vi "Get ROI Description String.vi"(8 "Error In":errorcluster, 9 "Contours":T2(array[cluster]), 11 "Global Rectangle":i32[](array[numeric])) -> (0 "Error Out":errorcluster, 3 "ROI Description String":string)   [LabVIEW 2021, in "Image.lvlib"]
uses:
  Image.lvlib
  Image ROI Type.ctl
  Math/Math.lvlib
  Strings/Strings.lvlib
panel:
  in  "Type":T1
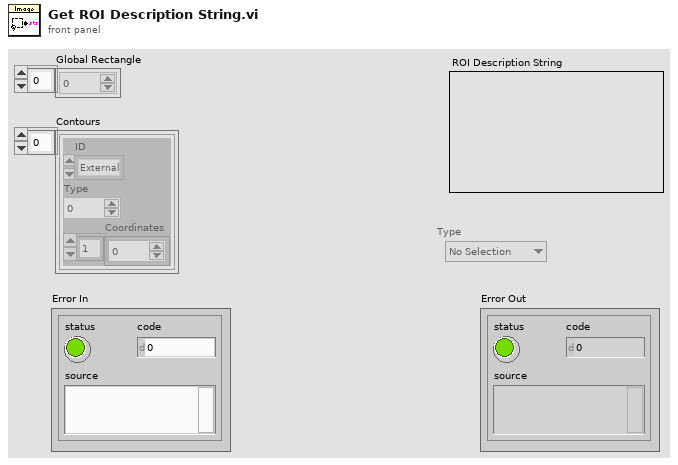
[diagram p1: front panel]
types:
  T1 = typedef "Image.lvlib/Image ROI Type.ctl" = enum16{"No Selection", "Point", "Line", "Rectangle", "Oval", "Polygon", "Freehand Region", "Annulus", "Unused2", "Unused3", "Broken Line", "Freehand Line", "Rotated Rectangle"}
  T2 = cluster{"ID":enum32{"External", "Internal"}, "Type":u32, "Coordinates":i32[]}[]
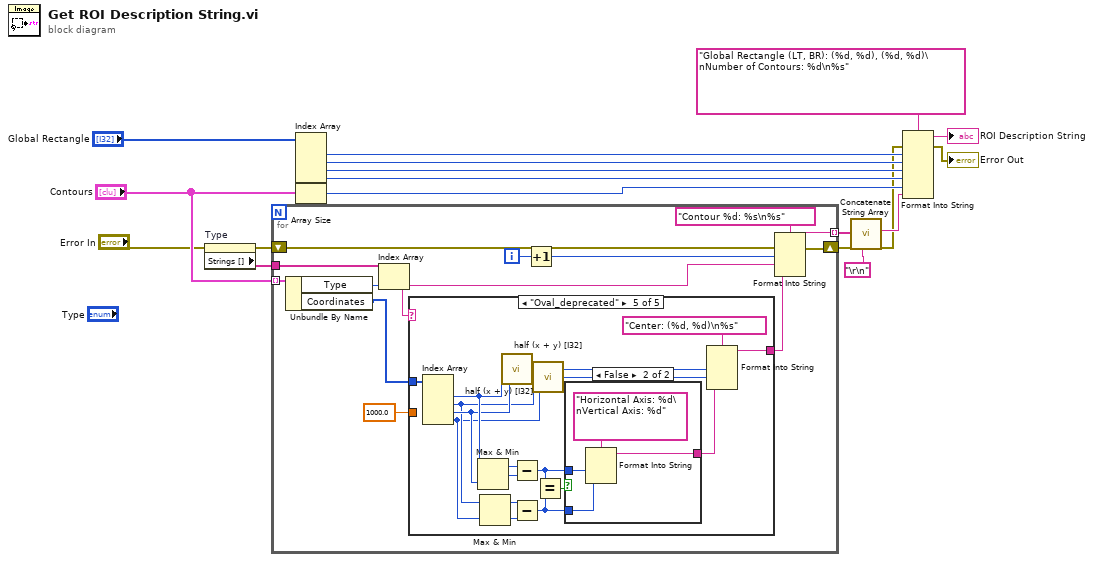
[diagram p0: block diagram]
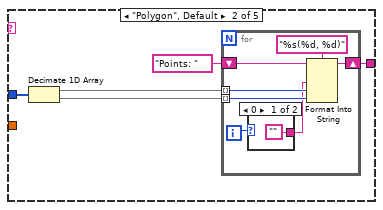
[diagram p3: hidden frame]
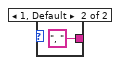
[diagram p4: hidden frame]
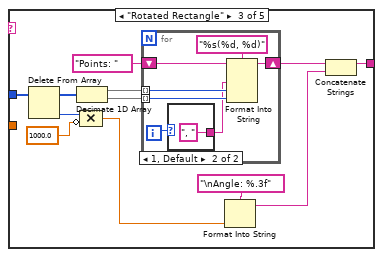
[diagram p5: hidden frame]
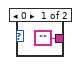
[diagram p6: hidden frame]
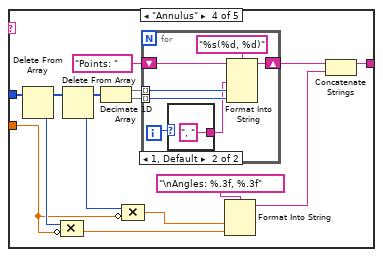
[diagram p7: hidden frame]
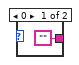
[diagram p8: hidden frame]
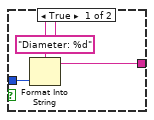
[diagram p9: hidden frame]
diagram:
  n1 = property on="Type" class="Enum (strict)"(error in="Error In") -> (error out=w1:errorcluster, "Strings []"=w5:string[])  [unwired: 1 in, 1 out]
  n2 = for {
    tunnel: "Contours" -> [w30] mode=indexing
    tunnel: w5 -> [w29]
    tunnel: [w25] -> w8 mode=indexing
    shift-right: [w19] -> w4
    shift-left: w1 -> [w20]
    i -> [w27]
    n3 = Unbundle By Name(w30) -> ("Type"=w23:u32, "Coordinates"=w21:i32[])
    n4 = Index Array(array=w29, index=w23) -> (element=w22:string)
    n5 = case shown="\"Oval_deprecated\"" w22 {
      tunnel: [_ w35 w50 w74 w106] -> w24
      tunnel: w21 -> [_ w34 w55 w79 w104]
      tunnel: 1000.0 ("value") -> [_ _ _ w67 _]
      frame "No Selection" {
      }
      frame "Polygon", Default {
        n6 = Decimate 1D Array(w34) -> (w33:i32[], w32:i32[])
        n7 = for {
          tunnel: w33 -> [w38] mode=indexing
          tunnel: w32 -> [w40] mode=indexing
          shift-right: [w41] -> w35
          shift-left: "Points: " -> [w42]
          i -> [w37]
          n8 = case shown="0" w37 {
            tunnel: ["" ", "] -> w36
            frame 0 {
            }
            frame 1, Default {
            }
          }
          n9 = Format Into String(format string="%s(%d, %d)", initial string=w42, w36, w38, w40) -> (resulting string=w41:string)  [unwired: 1 in, 1 out]
        }
      }
      frame "Rotated Rectangle" {
        n10 = Delete From Array(array=w55) -> (deleted portion=w49:i32, array with subset deleted=w51:i32[])  [unwired: 2 in]
        n11 = Decimate 1D Array(w51) -> (w54:i32[], w53:i32[])
        n12 = Compound Arithmetic op=MULTIPLY(w49, invert 1000.0 ("value")) -> (w46:dbl)
        n13 = for {
          tunnel: w54 -> [w59] mode=indexing
          tunnel: w53 -> [w61] mode=indexing
          shift-right: [w62] -> w56
          shift-left: "Points: " -> [w63]
          i -> [w58]
          n14 = case shown="1, Default" w58 {
            tunnel: ["" ", "] -> w57
            frame 0 {
            }
            frame 1, Default {
            }
          }
          n15 = Format Into String(format string="%s(%d, %d)", initial string=w63, w57, w59, w61) -> (resulting string=w62:string)  [unwired: 1 in, 1 out]
        }
        n16 = Format Into String(format string="\nAngle: %.3f", w46) -> (resulting string=w45:string)  [unwired: 2 in, 1 out]
        n17 = Concatenate Strings(w56, w45) -> (w50:string)
      }
      frame "Annulus" {
        n18 = Delete From Array(array=w79) -> (deleted portion=w73:i32, array with subset deleted=w75:i32[])  [unwired: 2 in]
        n19 = Compound Arithmetic op=MULTIPLY(w73, invert w67) -> (w69:dbl)
        n20 = Delete From Array(array=w75) -> (deleted portion=w68:i32, array with subset deleted=w70:i32[])  [unwired: 2 in]
        n21 = Decimate 1D Array(w70) -> (w78:i32[], w77:i32[])
        n22 = Compound Arithmetic op=MULTIPLY(w68, invert w67) -> (w66:dbl)
        n23 = for {
          tunnel: w78 -> [w83] mode=indexing
          tunnel: w77 -> [w85] mode=indexing
          shift-right: [w86] -> w80
          shift-left: "Points: " -> [w87]
          i -> [w82]
          n24 = case shown="1, Default" w82 {
            tunnel: ["" ", "] -> w81
            frame 0 {
            }
            frame 1, Default {
            }
          }
          n25 = Format Into String(format string="%s(%d, %d)", initial string=w87, w81, w83, w85) -> (resulting string=w86:string)  [unwired: 1 in, 1 out]
        }
        n26 = Format Into String(format string="\nAngles: %.3f, %.3f", w66, w69) -> (resulting string=w71:string)  [unwired: 2 in, 1 out]
        n27 = Concatenate Strings(w80, w71) -> (w74:string)
      }
      frame "Oval_deprecated" {
        n28 = Index Array(array=w104) -> (element #1=w101:i32, element #2=w97:i32, element #3=w100:i32, element #4=w96:i32)  [unwired: 4 in]
        n29 = Max & Min(x=w101, y=w100) -> (max(x,y)=w99:i32, min(x,y)=w98:i32)
        n30 = Max & Min(x=w97, y=w96) -> (max(x,y)=w95:i32, min(x,y)=w94:i32)
        n31 = call "half (x + y) [I32].vi"("y"=w100, "x"=w101) -> ("(x+y)/2"=w103:i32)  [unwired: 4 in]
        n32 = Subtract(x=w99, y=w98) -> (x-y=w92:i32)
        n33 = Subtract(x=w95, y=w94) -> (x-y=w90:i32)
        n34 = call "half (x + y) [I32].vi"("y"=w96, "x"=w97) -> ("(x+y)/2"=w102:i32)  [unwired: 4 in]
        n35 = Equal?(x=w92, y=w90) -> (x = y?=w93:bool)
        n36 = case shown="False" w93 {
          tunnel: w92 -> [w109 w113]
          tunnel: [w107 w111] -> w91
          tunnel: w90 -> [_ w110]
          frame True {
            n37 = Format Into String(format string="Diameter: %d", w109) -> (resulting string=w107:string)  [unwired: 2 in, 1 out]
          }
          frame False {
            n38 = Format Into String(format string="Horizontal Axis: %d\nVertical Axis: %d", w113, w110) -> (resulting string=w111:string)  [unwired: 2 in, 1 out]
          }
        }
        n39 = Format Into String(format string="Center: (%d, %d)\n%s", w103, w102, w91) -> (resulting string=w106:string)  [unwired: 2 in, 1 out]
      }
    }
    n40 = Increment(x=w27) -> (x+1=w26:i32)
    n41 = Format Into String(format string="Contour %d: %s\n%s", error in=w20, w26, w22, w24) -> (resulting string=w25:string, error out=w19:errorcluster)  [unwired: 1 in]
  }
  n42 = Index Array(array="Global Rectangle") -> (element #1=w11:i32, element #2=w12:i32, element #3=w13:i32, element #4=w14:i32)  [unwired: 4 in]
  n43 = Array Size(array="Contours") -> (size(s)=w15:i32)
  n44 = call "Concatenate String Array.vi"("Separator (TAB)"="\r\n", "String Array"=w8) -> ("Formatted String"=w16:string)  [unwired: 9 in]
  n45 = Format Into String(format string="Global Rectangle (LT, BR): (%d, %d), (%d, %d)\nNumber of Contours: %d\n%s", error in=w4, w11, w12, w13, w14, w15, w16) -> (resulting string=→"ROI Description String":string, error out=→"Error Out":errorcluster)  [unwired: 1 in]
